vi "calculate_msg_length.vi"(10 "message":string) -> (2 "length":string)   [LabVIEW 2018]
doc: "Create a byte string representing message length (number of characters in the command, must be in range 0 to 57,800), not including checksum or length bytes, to be included in the command packet."
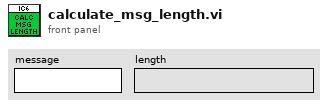
[diagram p1: front panel]
types:
  T1 = enum16{"big-endian, network order", "native, host order", "little-endian"}
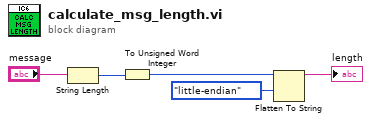
[diagram p0: block diagram]
diagram:
  n1 = String Length(string="message") -> (length=w3:i32)
  n2 = To Unsigned Word Integer(number=w3) -> (unsigned 16bit integer=w1:u16)
  n3 = Flatten To String(anything=w1, byte order (0:big-endian, network order)=T1."little-endian") -> (data string=→"length":string)  [unwired: 2 in, 2 out]
